vi "Build Cluster JSON.vi"(10 "Consumer?":bool, 11 "Cluster":variant) -> (3 "Array":T1[](array[typedef]))   [LabVIEW 2023, in "Utilities.lvlib"]
uses:
  Utilities.lvlib
  Channel.ctl
panel:
  in  "Channel":T1
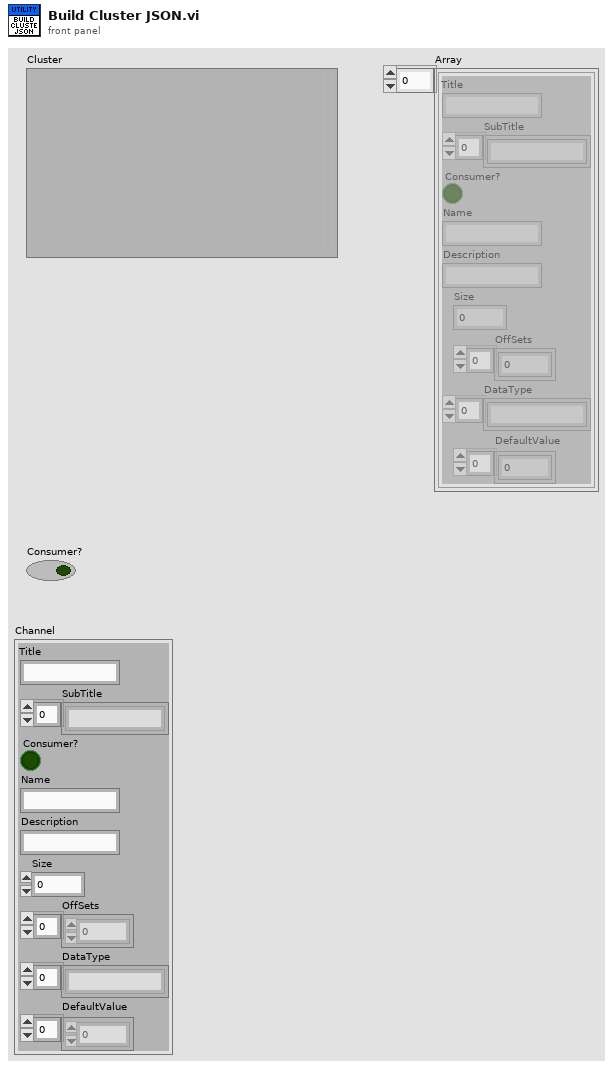
[diagram p1: front panel]
types:
  T1 = typedef "Utilities.lvlib/Channel.ctl" = cluster{"Title":string, "SubTitle":string[], "Consumer?":bool, "Name":string, "Description":string, "Size":i32, "OffSets":i32[], "DataType":string[], "DefaultValue":dbl[]}
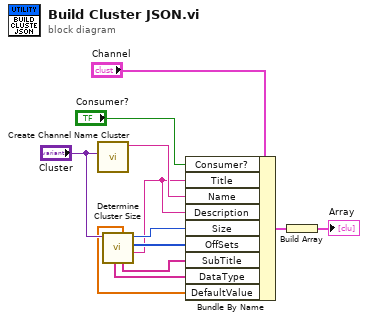
[diagram p0: block diagram]
diagram:
  n1 = call "Create Channel Name Cluster.vi"("Cluster"="Cluster") -> ("Data Channel Name"=w2:string)  [unwired: 9 in, 1 out]
  n2 = call "Determine Cluster Size.vi"("Variant"="Cluster") -> ("Title"=w1:string, "Offsets"=w11:i32[], "Total Size"=w12:i32, "SubChannelTitle"=w10:string[], "DefaultValues"=w3:dbl[], "DataType"=w9:string[])  [unwired: 4 in, 1 out]
  n3 = Bundle By Name(cluster="Channel", "Consumer?"="Consumer?", "Title"=w1, "Name"=w2, "Description"=w1, "Size"=w12, "OffSets"=w11, "SubTitle"=w10, "DataType"=w9, "DefaultValue"=w3) -> (w5:T1)
  n4 = Build Array(w5) -> (→"Array":T1[])
